vi "newsubvi Robot GoTo Park.vi"(0 "VISA In":refnum<visa-resource-name>) -> (1 "VISA Out":refnum<visa-resource-name>, 2 "error out":errorcluster)   [LabVIEW 2012]
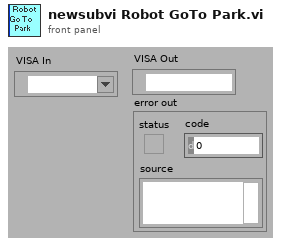
[diagram p1: front panel]
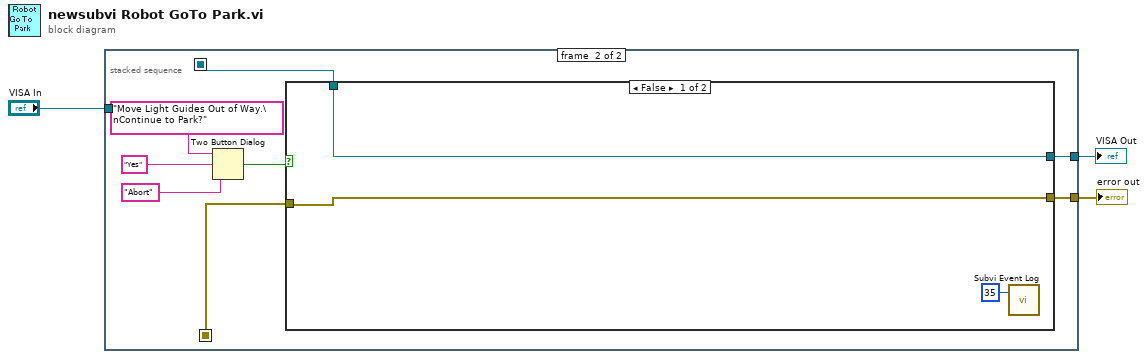
[diagram p0: block diagram]
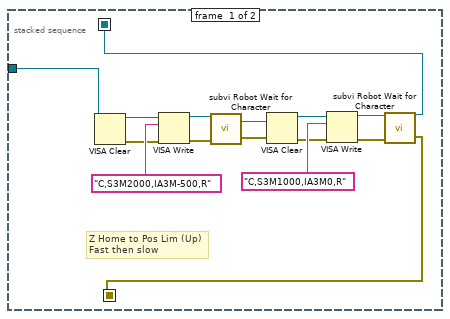
[diagram p2: hidden frame]
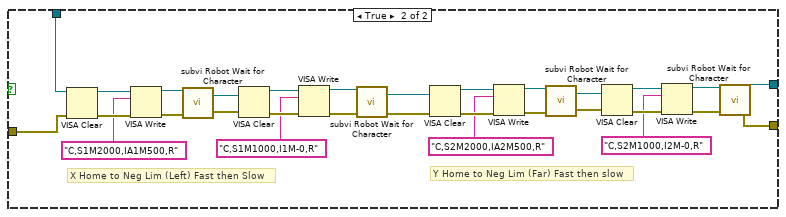
[diagram p3: hidden frame]
diagram:
  n1 = stacked-sequence {
    seq-local: [w5 _] -> [_ w22]
    seq-local: [w4 _] -> [_ w21]
    tunnel: "VISA In" -> [w18 _]
    tunnel: [_ w20] -> w2
    tunnel: [_ w19] -> w1
    frame #0 {
      # "Z Home to Pos Lim (Up)\nFast then slow"
      n2 = VISA Clear(VISA resource name=w18) -> (VISA resource name out=w17:refnum<visa-resource-name>, error out=w15:errorcluster)  [unwired: 1 in]
      n3 = VISA Write(VISA resource name=w17, write buffer="C,S3M2000,IA3M-500,R" ("Text to Send"), error in (no error)=w15) -> (VISA resource name out=w14:refnum<visa-resource-name>, error out=w13:errorcluster)  [unwired: 1 out]
      n4 = call "subvi Robot Wait for Character.vi"("error in"=w13, "VISA In"=w14) -> ("error out"=w11:errorcluster, "VISA Out"=w12:refnum<visa-resource-name>)
      n5 = VISA Clear(VISA resource name=w12, error in (no error)=w11) -> (VISA resource name out=w10:refnum<visa-resource-name>, error out=w8:errorcluster)
      n6 = VISA Write(VISA resource name=w10, write buffer="C,S3M1000,IA3M0,R" ("Text to Send"), error in (no error)=w8) -> (VISA resource name out=w7:refnum<visa-resource-name>, error out=w6:errorcluster)  [unwired: 1 out]
      n7 = call "subvi Robot Wait for Character.vi"("error in"=w6, "VISA In"=w7) -> ("error out"=w4:errorcluster, "VISA Out"=w5:refnum<visa-resource-name>)
    }
    frame #1 {
      n8 = Two Button Dialog(message="Move Light Guides Out of Way.\nContinue to Park?", 1:"Abort" ("F button name (\"Cancel\")"), 2:"Yes" ("T button name (\"OK\")")) -> (T button?=w23:bool)
      n9 = case shown="False" w23 {
        tunnel: w22 -> [w28 w59]
        tunnel: w21 -> [w27 w58]
        tunnel: [w28 w31] -> w20
        tunnel: [w27 w30] -> w19
        frame False {
          n10 = call "Subvi Event Log.vi"("EventNum"=u32 35) -> ()  [unwired: 1 in]
        }
        frame True {
          # "Y Home to Neg Lim (Far) Fast then slow"
          # "X Home to Neg Lim (Left) Fast then Slow"
          n11 = VISA Clear(VISA resource name=w59, error in (no error)=w58) -> (VISA resource name out=w57:refnum<visa-resource-name>, error out=w56:errorcluster)
          n12 = VISA Write(VISA resource name=w57, write buffer="C,S1M2000,IA1M500,R" ("Text to Send"), error in (no error)=w56) -> (VISA resource name out=w55:refnum<visa-resource-name>, error out=w54:errorcluster)  [unwired: 1 out]
          n13 = call "subvi Robot Wait for Character.vi"("error in"=w54, "VISA In"=w55) -> ("error out"=w52:errorcluster, "VISA Out"=w53:refnum<visa-resource-name>)
          n14 = VISA Clear(VISA resource name=w53, error in (no error)=w52) -> (VISA resource name out=w51:refnum<visa-resource-name>, error out=w50:errorcluster)
          n15 = VISA Write(VISA resource name=w51, write buffer="C,S1M1000,I1M-0,R" ("Text to Send"), error in (no error)=w50) -> (VISA resource name out=w49:refnum<visa-resource-name>, error out=w48:errorcluster)  [unwired: 1 out]
          n16 = call "subvi Robot Wait for Character.vi"("error in"=w48, "VISA In"=w49) -> ("error out"=w34:errorcluster, "VISA Out"=w35:refnum<visa-resource-name>)
          n17 = VISA Clear(VISA resource name=w35, error in (no error)=w34) -> (VISA resource name out=w45:refnum<visa-resource-name>, error out=w44:errorcluster)
          n18 = VISA Write(VISA resource name=w45, write buffer="C,S2M2000,IA2M500,R" ("Text to Send"), error in (no error)=w44) -> (VISA resource name out=w43:refnum<visa-resource-name>, error out=w42:errorcluster)  [unwired: 1 out]
          n19 = call "subvi Robot Wait for Character.vi"("error in"=w42, "VISA In"=w43) -> ("error out"=w40:errorcluster, "VISA Out"=w41:refnum<visa-resource-name>)
          n20 = VISA Clear(VISA resource name=w41, error in (no error)=w40) -> (VISA resource name out=w39:refnum<visa-resource-name>, error out=w38:errorcluster)
          n21 = VISA Write(VISA resource name=w39, write buffer="C,S2M1000,I2M-0,R" ("Text to Send"), error in (no error)=w38) -> (VISA resource name out=w37:refnum<visa-resource-name>, error out=w36:errorcluster)  [unwired: 1 out]
          n22 = call "subvi Robot Wait for Character.vi"("error in"=w36, "VISA In"=w37) -> ("error out"=w30:errorcluster, "VISA Out"=w31:refnum<visa-resource-name>)
        }
      }
    }
  }
  "VISA Out" <- w2
  "error out" <- w1
